vi "MCCMSG Get Scope Signal LPF.vi"(8 "error in (no error)":errorcluster, 9 "pnError":i32, 10 "pdLPF":dbl, 11 "hMCCmsg":i32) -> (0 "error out":errorcluster, 1 "pnError out":i32, 2 "pdLPF out":dbl, 3 "function return":i32)   [LabVIEW 2012, in "MultiClamp 700B Controls.lvlib" / "AxMultiClampMsg.lvlib"]
doc: "AXMCCMSG BOOL WINAPI MCCMSG_GetScopeSignalLPF(HMCCMSG hMCCmsg, double *pdLPF, int *pnError);"
uses:
  AxMultiClampMsg.lvlib
  AxMultiClampMsg.dll
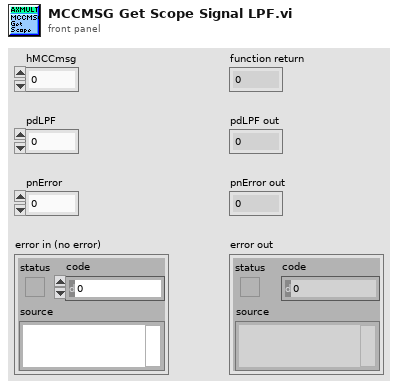
[diagram p1: front panel]
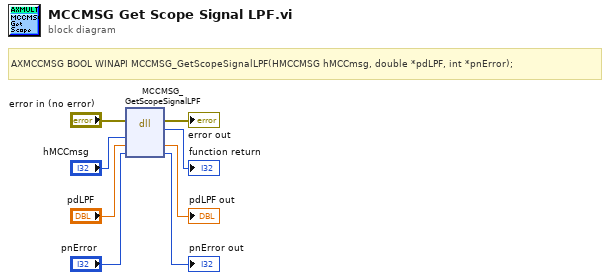
[diagram p0: block diagram]
diagram:
  # "AXMCCMSG BOOL WINAPI MCCMSG_GetScopeSignalLPF(HMCCMSG hMCCmsg, double *pdLPF, int *pnError);"
  n1 = dll-call lib="C:/Users/LAA12/Desktop/Rita/Multiclamp 700B VIs/AxMultiClampMsg/AxMultiClampMsg.*" fn="MCCMSG_GetScopeSignalLPF"(error in="error in (no error)", "hMCCmsg"="hMCCmsg", "pdLPF"="pdLPF", "pnError"="pnError") -> (error out=→"error out":errorcluster, →"function return":i32, "pdLPF"=→"pdLPF out":dbl, "pnError"=→"pnError out":i32)  [unwired: 3 in, 1 out]
